vi "Set Up DB for Testing.vi"(7 "Additional Set Up Commands":string, 8 "Error In (no error)":errorcluster, 10 "Test DB Set Up Command":string, 11 "SQLite DB Operator In":refnum<class "SQLite DB Operator.lvclass">) -> (0 "Error Out":errorcluster, 2 "SQLite Connection":refnum<class "Connection.lvclass">, 3 "SQLite DB Operator Out":refnum<class "SQLite DB Operator.lvclass">)   [LabVIEW 2023]
uses:
  Clasess/SQLite DB Operator/SQLite DB Operator.lvclass
  <vilib>/drjdpowell/SQLite Library/SQL Connection/Connection.lvclass
  Clasess/SQLite DB Operator/SQLite DB Operator.lvclass/SQLite DB Operator.ctl
  <vilib>/drjdpowell/SQLite Library/SQL Connection/Execute SQL (No results).vi
  <vilib>/drjdpowell/SQLite Library/SQLite.lvlib
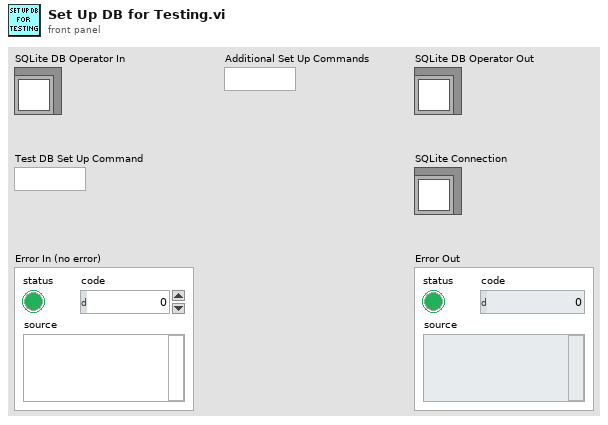
[diagram p1: front panel]
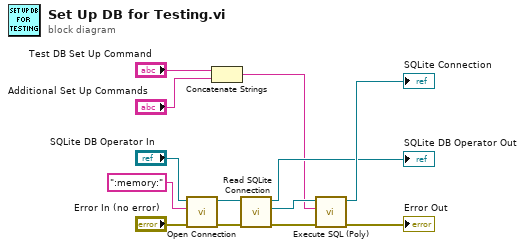
[diagram p0: block diagram]
diagram:
  n1 = call-dynamic "Open Connection.vi"("Error In (no error)"="Error In (no error)", "DB Connection String/Path"=":memory:" ("db file"), "SQLite DB Operator In"="SQLite DB Operator In") -> ("Error Out"=w11:errorcluster, "SQLite DB Operator Out"=w5:refnum<class "SQLite DB Operator.lvclass">)  [unwired: 7 in]
  n2 = Concatenate Strings("Test DB Set Up Command", "Additional Set Up Commands") -> (w2:string)
  n3 = call "Read SQLite Connection.vi"("Error In (no error)"=w11, "SQLite DB Operator In"=w5) -> ("Error Out"=w6:errorcluster, "SQLite.lvlib:Connection"=w7:refnum<class "Connection.lvclass">, "SQLite DB Operator out"=→"SQLite DB Operator Out":refnum<class "SQLite DB Operator.lvclass">)  [unwired: 7 in]
  n4 = call-poly <vilib>:"Execute SQL (Poly).vi"("error in (no error)"=w6, "SQL"=w2, "SQLite Connection in"=w7) -> ("error out"=→"Error Out":errorcluster, "SQLite Connection"=→"SQLite Connection":refnum<class "Connection.lvclass">)  [unwired: 7 in]
